vi "Read Measurement Osciloscope.vi"(8 "error in (no error)":errorcluster, 10 "Read Measurement In":T1={"TEKTRONIX- READ-IN"={"Channel (1: Channel 1)"=1, "Measurement Type (0: Frequency)"=0}, "EDU-X-1200A- READ-IN"={"Slope Type (0: Positive)"=0, "Measurement Type (0: Peak-Peak)"=0, "Occurrence Value (1)"=1, "Vertical Cross Value (0)"=0.0}} {"EDU-X-1200A- READ-IN"."Measurement Type (0: Peak-Peak)" items=["Peak-Peak", "Maximum", "Minimum", "Amplitude", "Top", "Base", "Overshoot", "Preshoot", "Average - N Cycles", "Average - Full Screen", "DC RMS - N Cycles", "DC RMS - Full Screen", "AC RMS - N Cycles", "AC RMS - Full Screen (Std Dev)", "Ratio", "Period", "Frequency", "Counter", "+Width", "-Width", "Burst Width", "Duty Cycle", "Rise Time", "Fall Time", "Delay", "Phase", "X minY", "X maxY", "Positive Pulse Count", "Negative Pulse Count", "Raising Edge Count", "Falling Edge Count", "Area - N Cycle", "Area - Full Screen", "Nth Edge Time", "Nth Edge Cross Level Time"]; "EDU-X-1200A- READ-IN"."Slope Type (0: Positive)" items=["Positive", "Negative"]; "TEKTRONIX- READ-IN"."Measurement Type (0: Frequency)" items=["Frequency", "Mean", "Period", "Pulse Duty", "Peak to Peak", "Cycle RMS", "Minimum", "Maximum", "Rise Time", "Fall Time", "Positive Width", "Negative Width", "Amplitude", "Cycle Mean", "High", "Low", "Negative Duty", "Positive Overshoot", "Negative Overshoot", "Cursor Mean", "Burst Width", "Positive Pulse Count", "Negative Pulse Count", "Rising Edge Count", "Falling Edge Count", "Area", "Cycle Area", "RMS", "Cursor RMS"]; "TEKTRONIX- READ-IN"."Channel (1: Channel 1)" items=["Channel 1"=1, "Channel 2"=2, "Channel 3"=3, "Channel 4"=4]}, 11 "EDU-X 1002A in":refnum<class "EDU-X 1002A.lvclass">) -> (0 "error out":errorcluster, 2 "Read measurement Out":T2, 3 "EDU-X 1002A out":refnum<class "EDU-X 1002A.lvclass">)   [LabVIEW 2020, in "EDU-X 1002A.lvclass"]
uses:
  EDU-X 1002A.lvclass
  TypeDefs/ReadMeasurementOut--cluster.ctl
  TypeDefs/ReadMeasurementIn--cluster.ctl
  EDU-X 1002A.lvclass/EDU-X 1002A.ctl
  <instrlib>/Agilent 2000 3000 X-Series/Public/Data/Read Measurement (Current Value).vi
  <instrlib>/Agilent 2000 3000 X-Series/Agilent 2000 3000 X-Series.lvlib
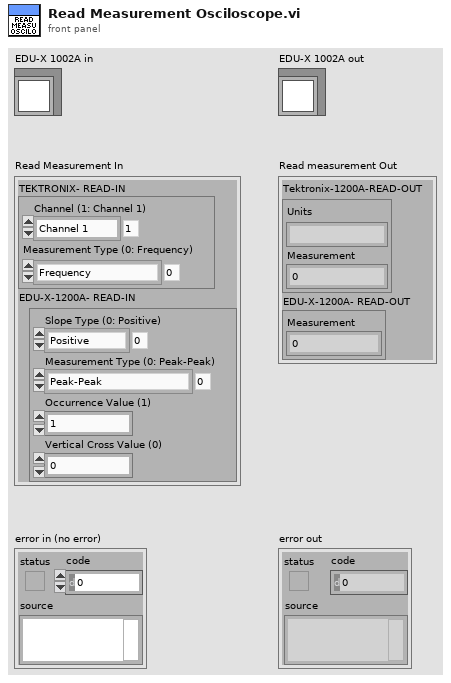
[diagram p1: front panel]
types:
  T1 = typedef "ReadMeasurementIn--cluster.ctl" = cluster{"TEKTRONIX- READ-IN":cluster{"Channel (1: Channel 1)":i32, "Measurement Type (0: Frequency)":i32}, "EDU-X-1200A- READ-IN":cluster{"Slope Type (0: Positive)":i32, "Measurement Type (0: Peak-Peak)":i32, "Occurrence Value (1)":i32, "Vertical Cross Value (0)":dbl}}
  T2 = typedef "ReadMeasurementOut--cluster.ctl" = cluster{"Tektronix-1200A-READ-OUT":cluster{"Units":string, "Measurement":dbl}, "EDU-X-1200A- READ-OUT":cluster{"Measurement":dbl}}
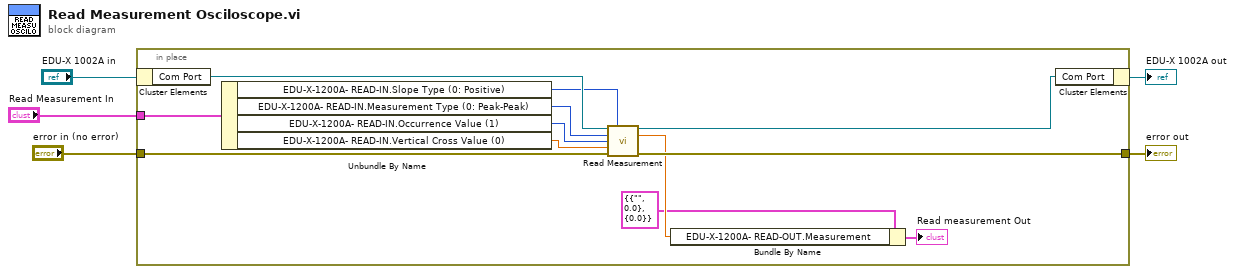
[diagram p0: block diagram]
diagram:
  n1 = in-place {
    in-place-border: "error in (no error)" -> [w11]
    in-place-border: "Read Measurement In" -> [w10]
    in-place-border: [w9] -> w1
    n2 = in-place-cluster #1("EDU-X 1002A in") -> ("Com Port"=w17:refnum<visa-resource-name>)
    n3 = Unbundle By Name(w10) -> ("EDU-X-1200A- READ-IN.Slope Type (0: Positive)"=w15:i32, "EDU-X-1200A- READ-IN.Measurement Type (0: Peak-Peak)"=w14:i32, "EDU-X-1200A- READ-IN.Occurrence Value (1)"=w13:i32, "EDU-X-1200A- READ-IN.Vertical Cross Value (0)"=w12:dbl)
    n4 = call-poly <instrlib>:"Read Measurement.vi"("VISA resource name"=w17, "Slope Type (0: Positive)"=w15, "Measurement Type (0: Peak-Peak)"=w14, "Occurrence Value (1)"=w13, "Vertical Cross Value (0)"=w12, "error in (no error)"=w11) -> ("VISA resource name out"=w16:refnum<visa-resource-name>, "Result Value"=w8:dbl, "error out"=w9:errorcluster)  [unwired: 7 in]
    n5 = Bundle By Name(cluster=T2 {"Tektronix-1200A-READ-OUT"={"Units"="", "Measurement"=0.0}, "EDU-X-1200A- READ-OUT"={"Measurement"=0.0}} ("Read measurement Out"), "EDU-X-1200A- READ-OUT.Measurement"=w8) -> (→"Read measurement Out":T2)
    n6 = in-place-cluster #1("Com Port"=w16) -> (→"EDU-X 1002A out":refnum<class "EDU-X 1002A.lvclass">)
  }
  "error out" <- w1
